vi "SVI_SpeciesChecker.vi"(11 "Species in":string) -> (1 "Changed":bool, 3 "Species out":string)   [LabVIEW 2014]
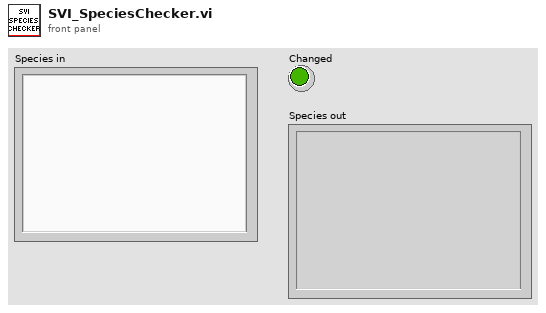
[diagram p1: front panel]
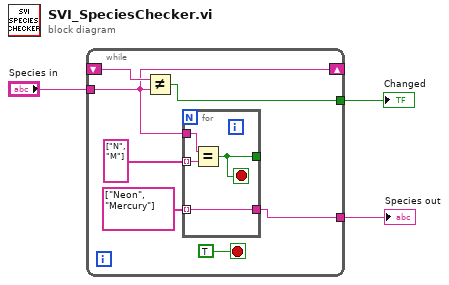
[diagram p0: block diagram]
diagram:
  n1 = while {
    shift-right: [w4] -> _
    shift-left: _ -> [w7]
    tunnel: [w9] -> w2
    tunnel: [w5] -> w3
    tunnel: "Species in" -> [w4]
    stop <- TRUE stop-if-true
    n2 = Not Equal?(x=w7, y=w4) -> (x != y?=w9:bool)
    n3 = for {
      tunnel: w4 -> [w14]
      tunnel: string[] ["N", "M"] -> [w12] mode=indexing
      tunnel: [w13] -> _
      tunnel: string[] ["Neon", "Mercury"] -> [w11] mode=indexing
      tunnel: [w11] -> w5
      stop <- w13 stop-if-true
      n4 = Equal?(x=w14, y=w12) -> (x = y?=w13:bool)
    }
  }
  "Species out" <- w3
  "Changed" <- w2
